vi "Philosofers_console.vi"() -> ()   [LabVIEW 2015]
uses:
  endallprocess.ctl
panel:
  out "280-309":bool[](array[boolean])
  out "240-279":bool[](array[boolean])
  out "210-239":bool[](array[boolean])
  out "180-209":bool[](array[boolean])
  out "150-179":bool[](array[boolean])
  out "120-149":bool[](array[boolean])
  out "90-119":bool[](array[boolean])
  out "60-89":bool[](array[boolean])
  out "30-59":bool[](array[boolean])
  out "0-29":bool[](array[boolean])
  in  "stop":T1
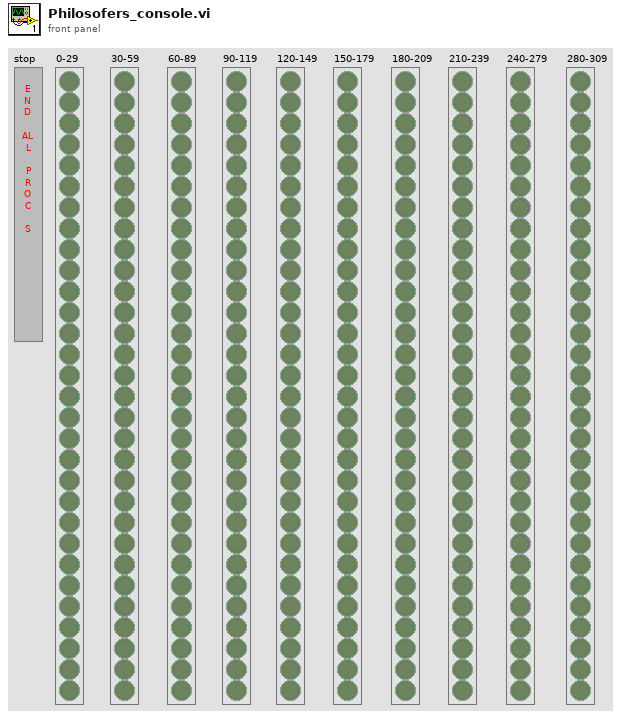
[diagram p1: front panel]
types:
  T1 = typedef "endallprocess.ctl" = bool
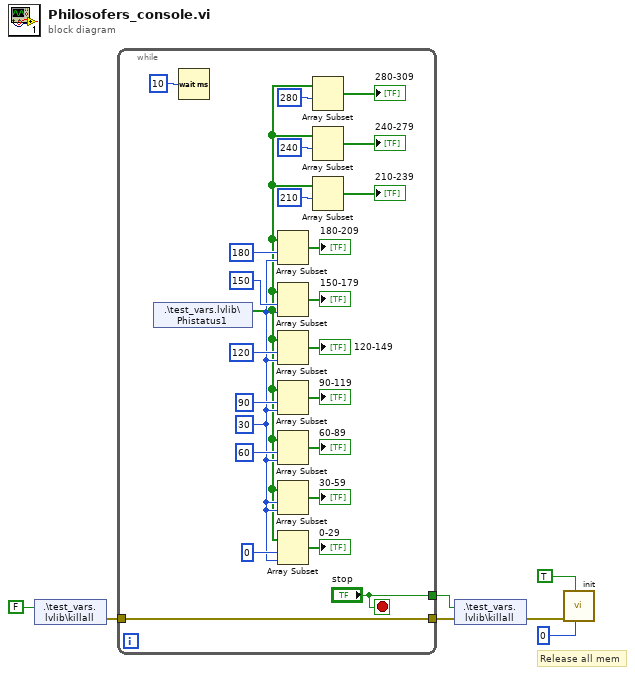
[diagram p0: block diagram]
diagram:
  # "Release all mem"
  n1 = shared-variable ".\\test_vars.lvlib\\killall"(FALSE ("killall")) -> (error out=w5:errorcluster)  [unwired: 1 in]
  n2 = while {
    tunnel: ["stop"] -> w7
    tunnel: w5 -> [w29]
    tunnel: [w29] -> w4
    stop <- "stop" stop-if-true
    w15 = 30 ("length")
    n3 = shared-variable ".\\test_vars.lvlib\\Phistatus1"() -> (w8:bool[])  [unwired: 1 in, 1 out]
    n4 = Wait (ms)(milliseconds to wait=u32 10) -> ()  [unwired: 1 out]
    n5 = Array Subset(array=w8, index=180, length=w15) -> (→"180-209":bool[])
    n6 = Array Subset(array=w8, index=150, length=w15) -> (→"150-179":bool[])
    n7 = Array Subset(array=w8, index=120, length=w15) -> (→"120-149":bool[])
    n8 = Array Subset(array=w8, index=90, length=w15) -> (→"90-119":bool[])
    n9 = Array Subset(array=w8, index=60, length=w15) -> (→"60-89":bool[])
    n10 = Array Subset(array=w8, index=w15, length=w15) -> (→"30-59":bool[])
    n11 = Array Subset(array=w8, index=0, length=w15) -> (→"0-29":bool[])
    n12 = Array Subset(array=w8, index=280) -> (→"280-309":bool[])  [unwired: 1 in]
    n13 = Array Subset(array=w8, index=240) -> (→"240-279":bool[])  [unwired: 1 in]
    n14 = Array Subset(array=w8, index=210) -> (→"210-239":bool[])  [unwired: 1 in]
  }
  n15 = shared-variable ".\\test_vars.lvlib\\killall"(w7, error in=w4) -> (error out=w3:errorcluster)
  n16 = call "init.vi"("Space size"=0, "Cleaneup"=TRUE, "error in (no error)"=w3) -> ()  [unwired: 8 in, 1 out]
